vi "run.vi"(8 "error in (no error)":errorcluster, 10 "Path":path, 11 "CameraSettingsViewer in":refnum<class "andorSettingsViewer.lvclass">) -> (0 "error out":errorcluster, 3 "CameraSettingsViewer out":refnum<class "andorSettingsViewer.lvclass">)   [LabVIEW 2011, in "Views.lvlib" / "Camera.lvlib" / "andorSettingsViewer.lvclass"]
uses:
  andorSettingsViewer.lvclass
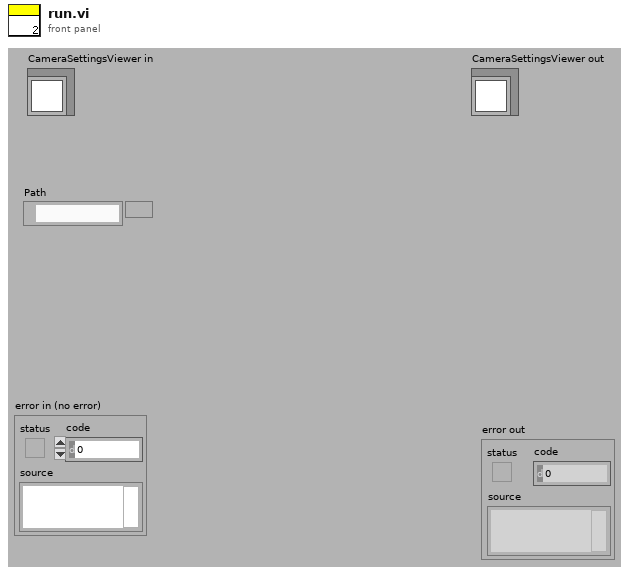
[diagram p1: front panel]
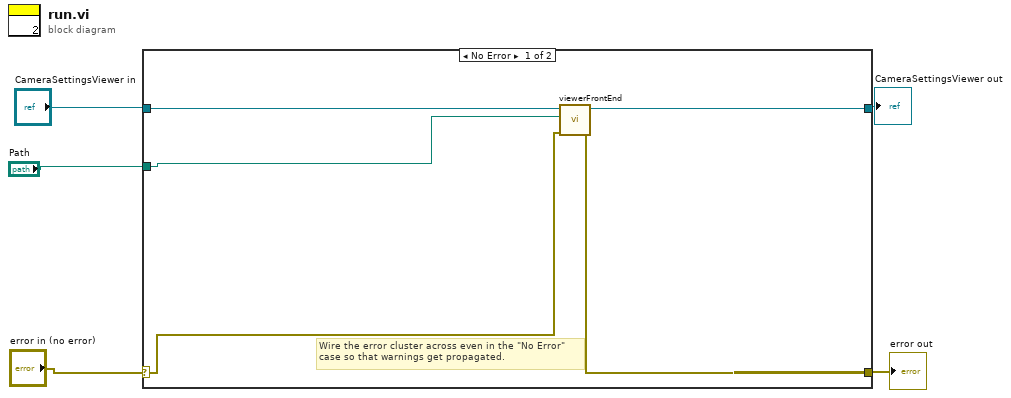
[diagram p0: block diagram]
diagram:
  n1 = case shown="No Error" "error in (no error)" {
    selector: "error in (no error)" -> [w6 w12]
    tunnel: [w9 w12] -> w4
    tunnel: [w10 w11] -> w1
    tunnel: "CameraSettingsViewer in" -> [w7 w11]
    tunnel: "Path" -> [w8 _]
    frame No Error {
      # "Wire the error cluster across even in the \"No Error\"\ncase so that warnings get propagated."
      n2 = call-dynamic "viewerFrontEnd.vi"("error in (no error)"=w6, "defaultPath"=w8, "CameraSettingsViewer in"=w7) -> ("error out"=w9:errorcluster, "CameraSettingsViewer out"=w10:refnum<class "andorSettingsViewer.lvclass">)  [unwired: 7 in]
    }
    frame Error {
    }
  }
  "CameraSettingsViewer out" <- w1
  "error out" <- w4
